vi "Instantiate.vi"(1 "vi ref":refnum<vi>) -> (0 "vi ref":refnum<vi>)   [LabVIEW 2020, in "Tag-t'input_params.ctl'.lvlib"]
doc: "Creates and initializes the data structure that supports the channel at run time."
uses:
  <extravilib>/ChannelInstances/Tag-t'input_params.ctl'.lvlib
  <extravilib>/ChannelInstances/Tag-t'input_params.ctl'/ChannelOp.ctl
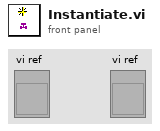
[diagram p1: front panel]
types:
  T1 = typedef "Tag-t'input_params.ctl'.lvlib/ChannelOp.ctl" = enum16{"init", "write", "read", "probe"}
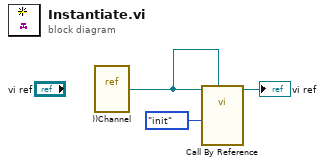
[diagram p0: block diagram]
diagram:
  n1 = vi-ref <extravilib>:"))Channel.vi"() -> (w2:refnum<vi>)
  n2 = call-by-ref "?"(reference=w2, "This VI"=w2, "channelOp"=ChannelOp."init") -> (reference out=→"vi ref":refnum<vi>)  [unwired: 5 in, 7 out]
